vi "data_out.vi"(8 "error in (no error)":errorcluster, 11 "Analog_Input (in)":refnum<class "Analog_Input.lvclass">) -> (0 "error out":errorcluster, 2 "AI data string":string, 3 "Analog_Input":refnum<class "Analog_Input.lvclass">)   [LabVIEW 2013, in "Analog_Input.lvclass"]
uses:
  Analog_Input.lvclass
  Analog_Input.lvclass/Analog_Input.ctl
  Globals.vi
  TCP_IP/TCP_IP.lvclass
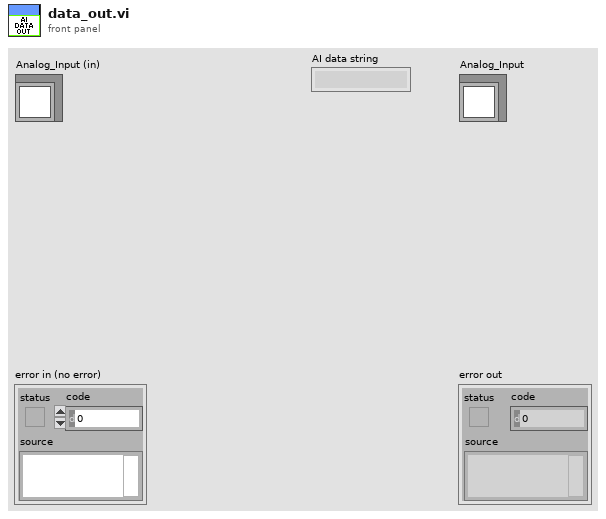
[diagram p1: front panel]
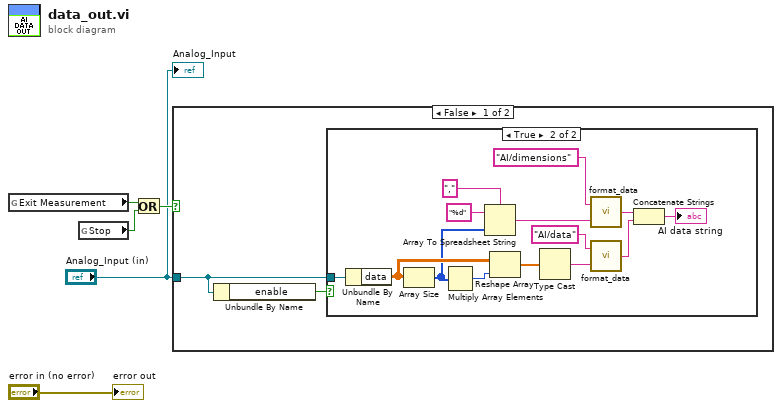
[diagram p0: block diagram]
diagram:
  n1 = global read "Globals.vi" "Exit Measurement"() -> (w5:bool)
  n2 = global read "Globals.vi" "Stop"() -> (w4:bool)
  n3 = Or(x=w5, y=w4) -> (x .or. y?=w3:bool)
  n4 = case shown="False" w3 {
    tunnel: "Analog_Input (in)" -> [w6 _]
    frame False {
      n5 = Unbundle By Name(w6) -> ("enable"=w7:bool)
      n6 = case shown="True" w7 {
        tunnel: w6 -> [_ w21]
        frame False {
        }
        frame True {
          n7 = Unbundle By Name(w21) -> ("data"=w12:dbl[][])
          n8 = Array Size(array=w12) -> (size(s)=w11:i32[])
          n9 = Multiply Array Elements(1:w11) -> (0:w13:i32)
          n10 = Array To Spreadsheet String(delimiter (Tab)=",", array=w11, 3:"%d" ("format string")) -> (spreadsheet string=w16:string)
          n11 = Reshape Array(w12, w13) -> (w10:dbl[])
          n12 = Type Cast(x=w10) -> (*(type *) &x=w9:string)  [unwired: 1 in]
          n13 = call "format_data.vi"("data"=w16, "name"="AI/dimensions") -> ("concatenated string"=w15:string)
          n14 = call "format_data.vi"("data"=w9, "name"="AI/data") -> ("concatenated string"=w14:string)
          n15 = Concatenate Strings(w15, w14) -> (→"AI data string":string)
        }
      }
    }
    frame True {
    }
  }
  "error out" <- "error in (no error)"
  "Analog_Input" <- "Analog_Input (in)"
